vi "test-globallog for register and unregister VI.vi"(8 "error in (no error)":errorcluster, 11 "TestCase in":refnum<class "testcase-globalLog.lvclass">) -> (0 "error out":errorcluster, 3 "TestCase out":refnum<class "testcase-globalLog.lvclass">)   [LabVIEW 2017, in "testcase-globalLog.lvclass"]
uses:
  testcase-globalLog.lvclass
  src/user.lib/_NEVSTOP/Communicable State Machine(CSM)/_Support/Typedef/_CSM_GlobalLog_MSG.ctl
  src/user.lib/_NEVSTOP/Communicable State Machine(CSM)/_Support/Typedef/_CSM_Response Source Message.ctl
  src/user.lib/_NEVSTOP/Communicable State Machine(CSM)/_Support/Typedef/_CSM_GlobalLog_MSG_TYPE.ctl
  <vilib>/addons/_JKI Toolkits/VI Tester/TestCase.llb/TestCase.lvclass
  src/user.lib/_NEVSTOP/Communicable State Machine(CSM)/Communicable State Machine.lvlib
  C:/Program Files (x86)/National Instruments/LabVIEW 2017/vi.lib/addons/_JKI Toolkits/VI Tester/TestCase.llb/TestCase.lvclass
panel:
  in  "Exit?":bool=TRUE
  out "State History":string
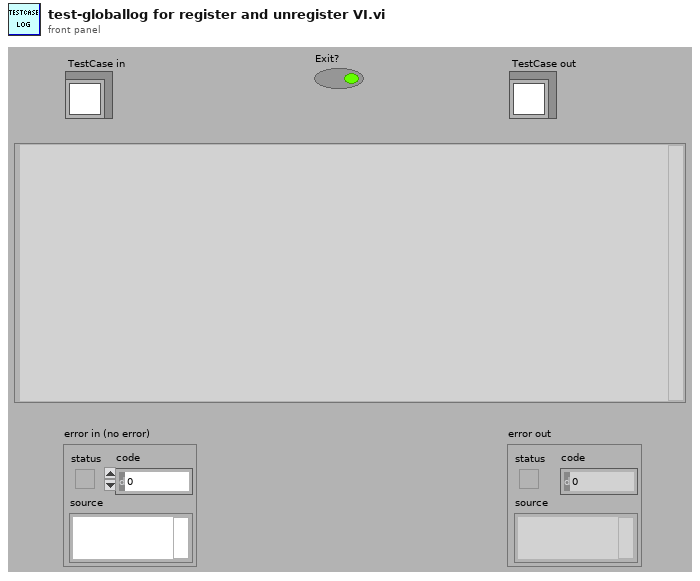
[diagram p1: front panel]
types:
  T1 = cluster{"threashold(#/s)":dbl, "Check Peroid(s)":dbl}
  T2 = typedef "Communicable State Machine.lvlib/_CSM_GlobalLog_MSG.ctl" = cluster{"Name (\"\" to Use UUID)":string, "Current State":string, "Arguments":string, "Source Message":T3, "Source Module":string, "Complete(T)/Start(F)":bool, "LogType":T4, "Time Stamp":timestamp}
  T3 = typedef "Communicable State Machine.lvlib/_CSM_Response Source Message.ctl" = cluster{"‘State":string, "’Arguments":string, "’Error":errorcluster}
  T4 = typedef "Communicable State Machine.lvlib/_CSM_GlobalLog_MSG_TYPE.ctl" = enum16{"User Log", "State Change", "Status", "Interrupt", "Register", "Unregister", "Error Log", "Module Created", "Module Destroyed"}
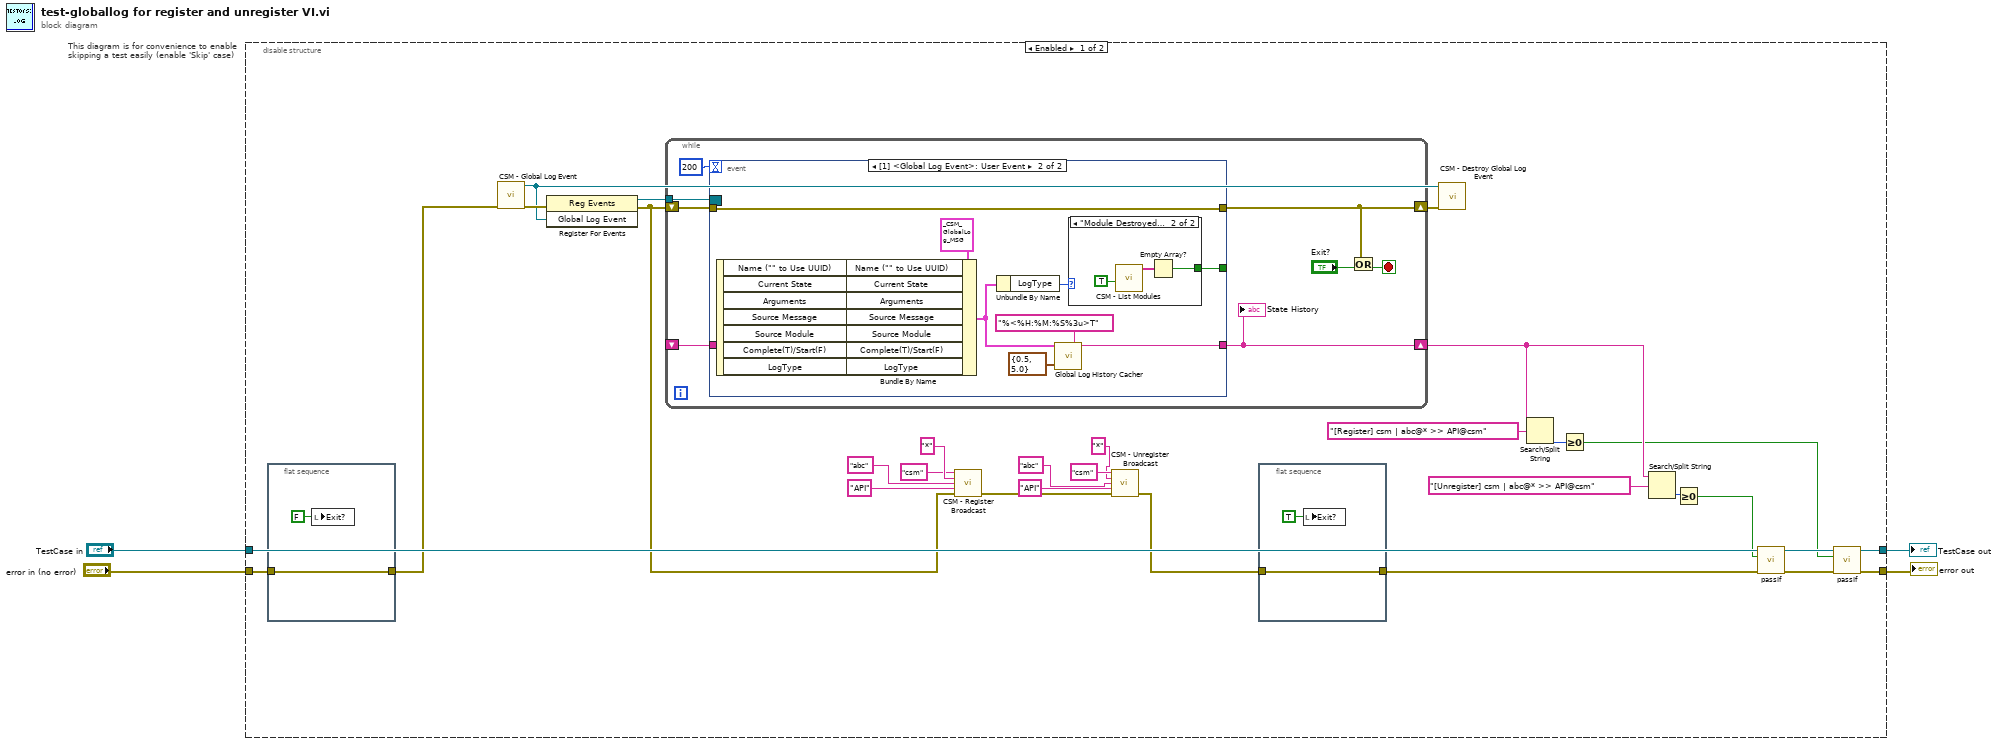
[diagram p0: block diagram]
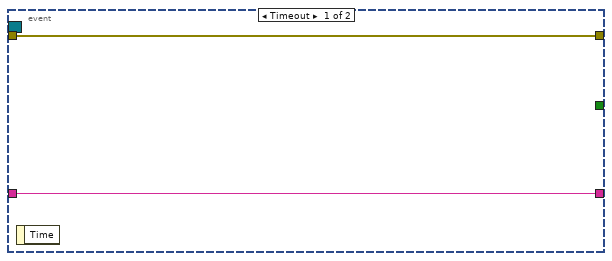
[diagram p2: hidden frame]
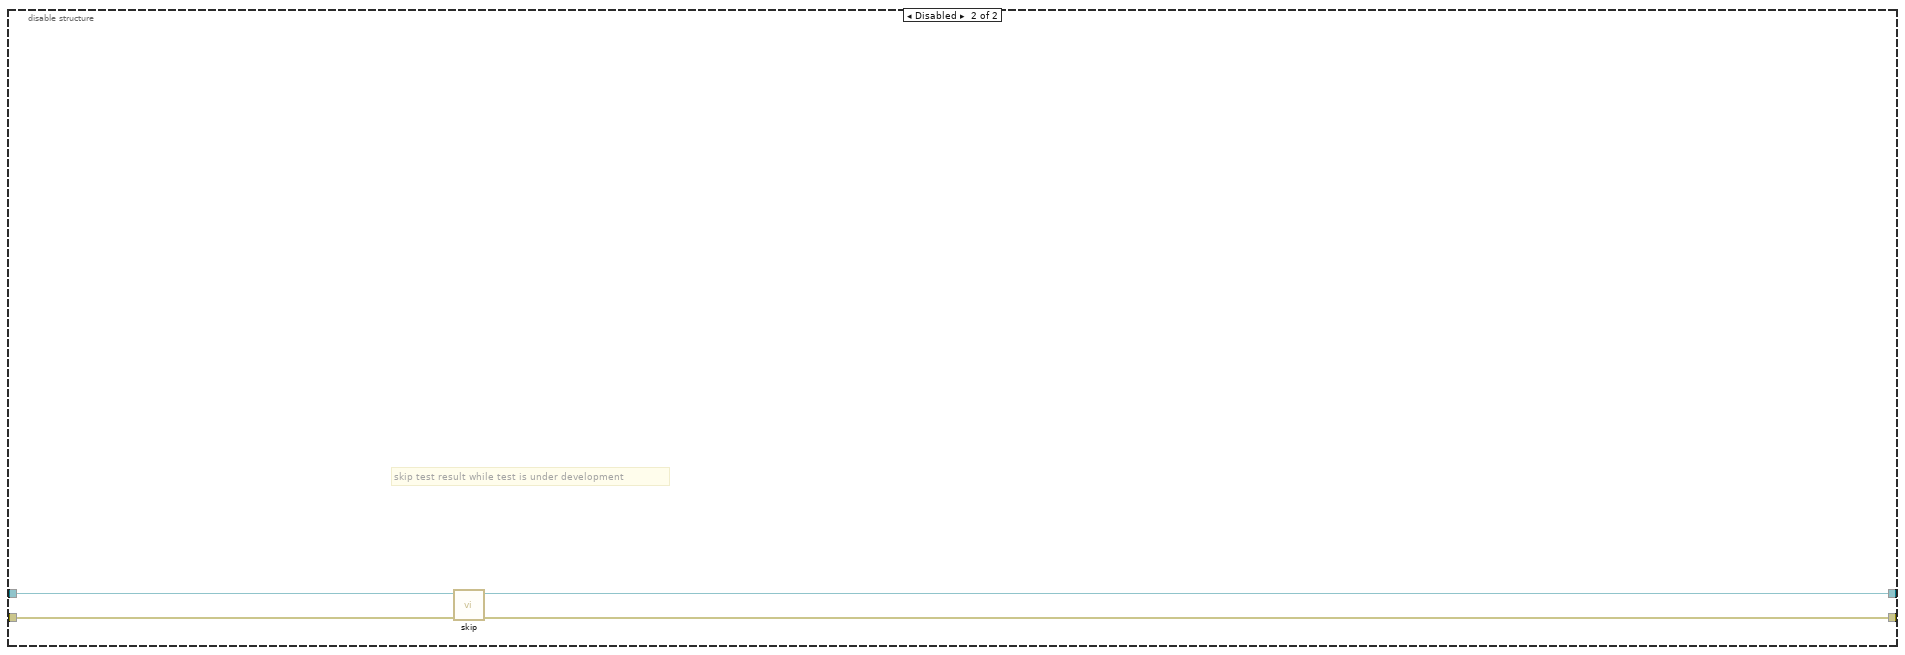
[diagram p4: hidden frame]
diagram:
  n1 = disable-structure "This diagram is for convenience to enable skipping a test easily (enable 'Skip' case)" shown="Enabled" {
    disable-tunnel: "TestCase in" -> [w34 w70]
    disable-tunnel: [w13 w68] -> w1
    disable-tunnel: [w14 w69] -> w3
    disable-tunnel: "error in (no error)" -> [w33 w67]
    frame Enabled {
      n2 = flat-sequence {
        tunnel: [w65] -> w24
        tunnel: w33 -> [w65]
        frame #0 {
          n3 = local write "Exit?"(FALSE ("Exit?")) -> ()
        }
      }
      n4 = call "CSM - Global Log Event.vi"("Error In"=w24) -> ("error out"=w27:errorcluster, "Global Log Event"=w25:refnum<user-event>)  [unwired: 9 in]
      n5 = register-events(error in=w27, w25) -> (reference out=w28:refnum<event-registration>, error out=w23:errorcluster)  [unwired: 1 in]
      n6 = while {
        tunnel: w28 -> [w42]
        shift-right: [w39] -> w26
        shift-left: w23 -> [w41]
        shift-right: [w37] -> w10
        shift-left: _ -> [w36]
        stop <- w40 stop-if-true
        n7 = event shown="[1] <Global Log Event>: User Event" {
          selector: w42 -> [_ _]
          dyn-events: _ -> [_ _]
          timeout: 200 -> [_ _]
          tunnel: w41 -> [w44 w59]
          tunnel: [w44 w59] -> w39
          tunnel: [_ w48] -> _
          tunnel: [w43 w45] -> w37
          tunnel: w36 -> [w43 _]
          event Timeout {
            n8 = event-data() -> ()  [unwired: 1 in, 1 out]
          }
          event User Event {
            n9 = event-data() -> ("Name (\"\" to Use UUID)"=w58:string, "Current State"=w57:string, "Arguments"=w56:string, "Source Message"=w55:T3, "Source Module"=w54:string, "Complete(T)/Start(F)"=w53:bool, "LogType"=w52:T4)  [unwired: 1 in]
            n10 = Bundle By Name(cluster=T2 {"Name (\"\" to Use UUID)"="", "Current State"="", "Arguments"="", "Source Message"={"‘State"="", "’Arguments"="", "’Error"={"status"=FALSE, "code"=0, "source"=""}}, "Source Module"="", "Complete(T)/Start(F)"=FALSE, "LogType"=enum."State Change", "Time Stamp"=timestamp(0 s since 1904-01-01)} ("Cross CSM Data"), "Name (\"\" to Use UUID)"=w58, "Current State"=w57, "Arguments"=w56, "Source Message"=w55, "Source Module"=w54, "Complete(T)/Start(F)"=w53, "LogType"=w52) -> (w50:T2)
            n11 = Unbundle By Name(w50) -> ("LogType"=w49:T4)
            n12 = call "Global Log History Cacher.vi"("Global Log Data"=w50, "Time Format String"="%<%H:%M:%S%3u>T" ("Time format string"), "Settings"=T1 {"threashold(#/s)"=0.5, "Check Peroid(s)"=5.0}) -> ("String Cache"=w45:string)  [unwired: 12 in]
            n13 = case shown="\"Module Destroyed\"" w49 {
              tunnel: [_ w60] -> w48
              frame "User Log", Default {
              }
              frame "Module Destroyed" {
                n14 = call "CSM - List Modules.vi"("With Nodes? (F)"=TRUE ("All?")) -> ("Module Names"=w62:string[])  [unwired: 9 in, 1 out]
                n15 = Empty Array?(array=w62) -> (empty?=w60:bool)
              }
            }
          }
        }
        "State History" <- w37
        n16 = Or(x=w39, y="Exit?") -> (x .or. y?=w40:bool)
      }
      n17 = call "CSM - Register Broadcast.vi"("CSM Name"="csm", "Source CSM Name (* as Default)"="*", "Trigger"="abc" ("CSM Name"), "API (If \"\", Same as Trigger)"="API" ("Status"), "Error In"=w23) -> ("error out"=w31:errorcluster)  [unwired: 9 in, 1 out]
      n18 = call "CSM - Unregister Broadcast.vi"("CSM Name"="csm", "Source CSM Name (* as Default)"="*", "Trigger"="abc" ("CSM Name"), "API (\"*\" as Default)"="API" ("Status"), "Error In"=w31) -> ("error out"=w30:errorcluster)  [unwired: 9 in, 1 out]
      n19 = flat-sequence {
        tunnel: [w63] -> w32
        tunnel: w30 -> [w63]
        frame #0 {
          n20 = local write "Exit?"(TRUE ("Exit?")) -> ()
        }
      }
      n21 = call "CSM - Destroy Global Log Event.vi"("Error In"=w26, "CSM Global Log Event"=w25) -> ()  [unwired: 9 in, 1 out]
      n22 = Search/Split String(string=w10, search string/char (-)="[Register] csm | abc@* >> API@csm") -> (offset of match=w8:i32)  [unwired: 1 in, 2 out]
      n23 = Greater Or Equal To 0?(x=w8) -> (x >= 0?=w5:bool)
      n24 = Search/Split String(string=w10, search string/char (-)="[Unregister] csm | abc@* >> API@csm") -> (offset of match=w7:i32)  [unwired: 1 in, 2 out]
      n25 = Greater Or Equal To 0?(x=w7) -> (x >= 0?=w6:bool)
      n26 = call-dynamic "passIf.vi"("error in (no error)"=w32, "pass"=w6, "TestCase in"=w34) -> ("error out"=w15:errorcluster, "TestCase out"=w12:refnum<class "testcase-globalLog.lvclass">)  [unwired: 7 in]
      n27 = call-dynamic "passIf.vi"("error in (no error)"=w15, "pass"=w5, "TestCase in"=w12) -> ("error out"=w14:errorcluster, "TestCase out"=w13:refnum<class "testcase-globalLog.lvclass">)  [unwired: 7 in]
    }
    frame Disabled {
      # "skip test result while test is under development"
      n28 = call <vilib>:"skip.vi"("error in (no error)"=w67, "TestCase in"=w70) -> ("error out"=w69:errorcluster, "TestCase out"=w68:refnum<class "testcase-globalLog.lvclass">)  [unwired: 8 in]
    }
  }
  "error out" <- w3
  "TestCase out" <- w1
